vi "load_most_recent_calibration_file.vi"(4 "error in":errorcluster, 6 "pattern":string="*wavenumber.csv", 7 "Path":path=path "csv") -> (0 "error out":errorcluster, 3 "wavenumber vector":dbl[](array[numeric]))   [LabVIEW 2017]
uses:
  <vilib>/Utility/file.llb/Read Delimited Spreadsheet (DBL).vi
panel:
  out "Waveform Graph":cluster{dbl, dbl, "first row":dbl[]}(graph)
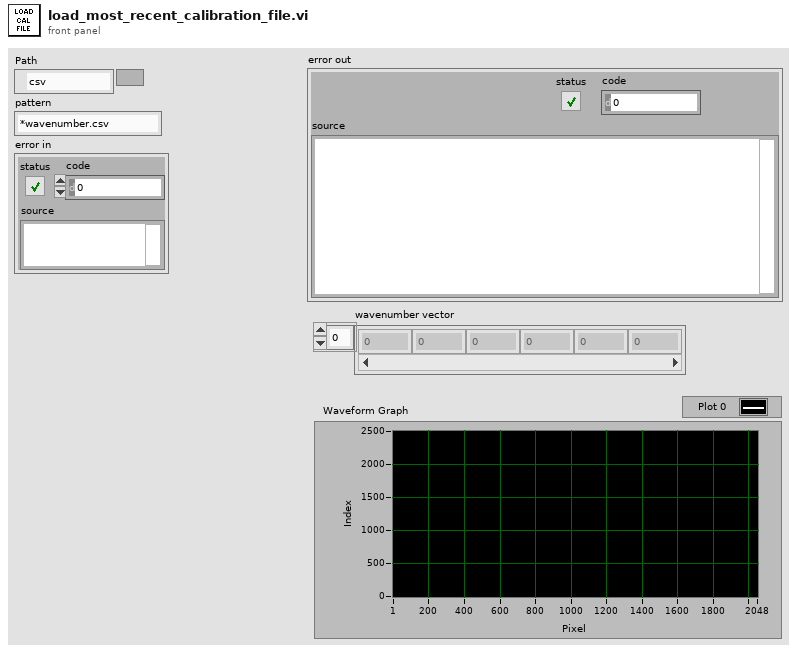
[diagram p1: front panel]
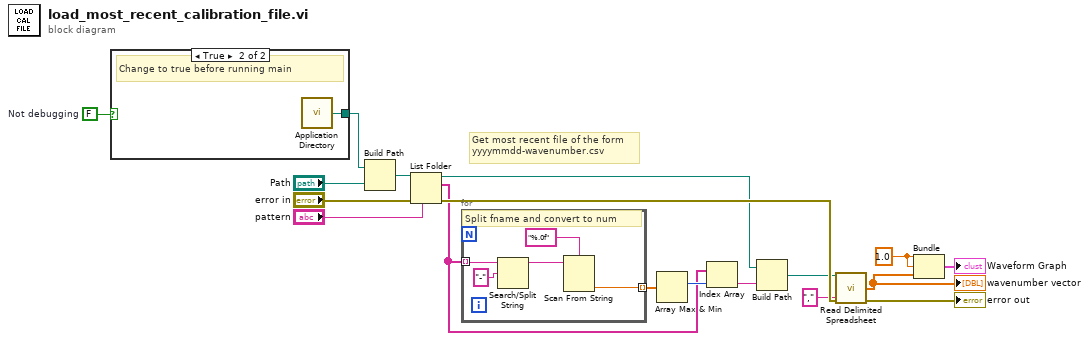
[diagram p0: block diagram]
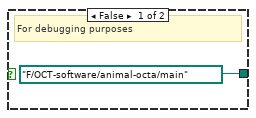
[diagram p2: hidden frame]
diagram:
  w3 = 1.0
  w11 = FALSE  # Not debugging
  # "Get most recent file of the form\nyyyymmdd-wavenumber.csv"
  n1 = case shown="True" w11 {
    tunnel: [path "F:/OCT-software/animal-octa/main" w20] -> w10
    frame False {
      # "For debugging purposes"
    }
    frame True {
      # "Change to true before running main"
      n2 = call <vilib>:"Application Directory.vi"() -> ("Application Directory"=w20:path)
    }
  }
  n3 = Build Path(base path=w10, name or relative path="Path") -> (appended path=w15:path)
  n4 = List Folder(path=w15, pattern="pattern", error in="error in") -> (path out=w6:path, filenames=w8:string[], error out=w17:errorcluster)  [unwired: 1 in, 1 out]
  n5 = for {
    tunnel: w8 -> [w24] mode=indexing
    tunnel: [w21] -> w9 mode=indexing
    # "Split fname and convert to num"
    n6 = Search/Split String(string=w24, search string/char (-)="-") -> (substring before match=w23:string)  [unwired: 1 in, 2 out]
    n7 = Scan From String(format string="%.0f", input string=w23) -> (output 1=w21:dbl)  [unwired: 3 in, 3 out]
  }
  n8 = Array Max & Min(array=w9) -> (max index (indices)=w16:i32)  [unwired: 3 out]
  n9 = Index Array(array=w8, index=w16) -> (element=w7:string)
  n10 = Build Path(base path=w6, name or relative path=w7) -> (appended path=w4:path)
  n11 = call-poly <vilib>:"Read Delimited Spreadsheet.vi"("file path (dialog if empty)"=w4, "error in (no error)"=w17, "delimiter (\\t)"="," ("delimiter (\\t)")) -> ("first row"=w2:dbl[], "error out"=→"error out":errorcluster)  [unwired: 7 in, 4 out]
  "wavenumber vector" <- w2
  n12 = Bundle(w3, w3, "first row"=w2) -> (→"Waveform Graph":cluster{dbl, dbl, "first row":dbl[]})  [unwired: 1 in]
